vi "InClassProb9-TankIO.vi"() -> ()   [LabVIEW 2017]
panel:
  out "AI3 Heater":dbl(slide) scale=0.0..100.0
  out "AI2 Tank 2":dbl(slide) scale=0.0..10.0
  out "AI1 Tank 1":dbl(slide) scale=0.0..10.0
  out "AI0 Main":dbl(slide) scale=0.0..10.0
  out "AI3":dbl
  out "AI2":dbl
  out "AI1":dbl
  out "AI0":dbl
  in  "Spare":bool
  in  "CM":bool
  in  "PM":bool
  in  "HT-01":bool
  in  "DV-02":bool
  in  "DV-01":bool
  in  "FV-02":bool
  in  "FV-01":bool
  out "data[1]":bool
  out "data[0]":bool
  in  "stop":bool
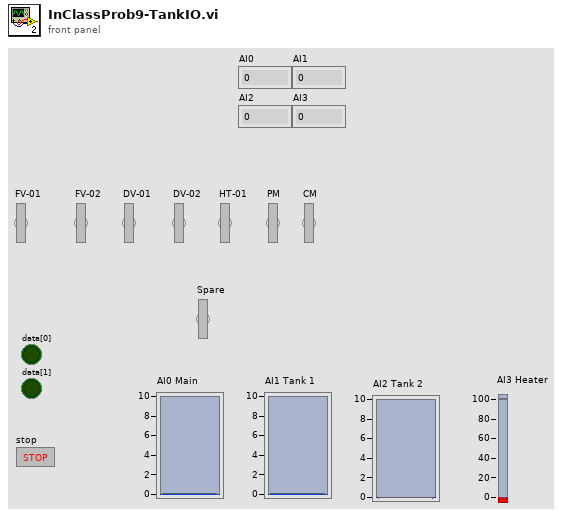
[diagram p1: front panel]
types:
  T1 = cluster{"data[0]":bool, "data[1]":bool, "data[2]":bool, "data[3]":bool, "data[4]":bool, "data[5]":bool, "data[6]":bool, "data[7]":bool, "data[8]":bool}
  T2 = cluster{"FV-01":bool, "FV-02":bool, "DV-01":bool, "DV-02":bool, "Spare":bool, "PM":bool, "CM":bool, "HT-01":bool}
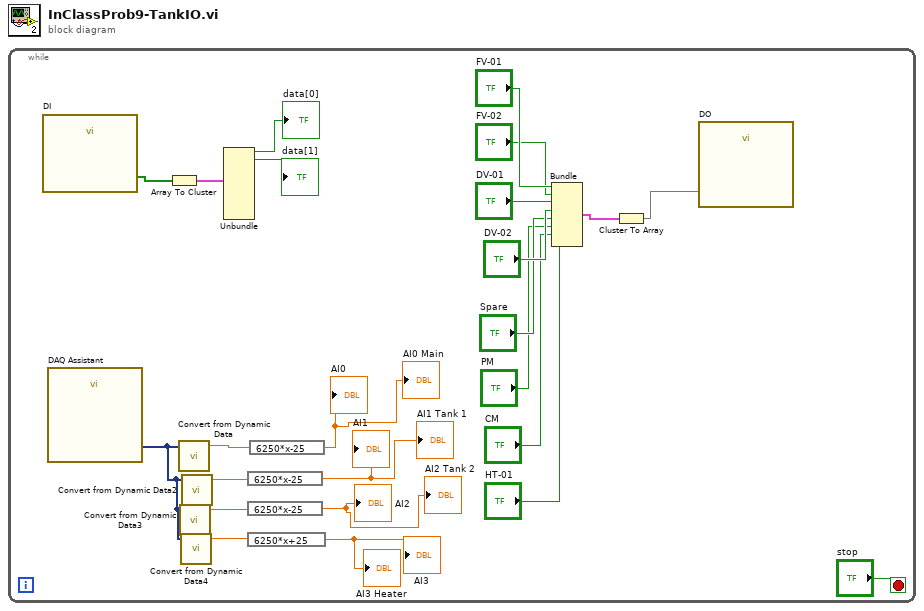
[diagram p0: block diagram]
diagram:
  n1 = while {
    stop <- "stop" stop-if-true
    n2 = call "DI"() -> ("data"=w23:bool[])  [unwired: 17 in, 2 out]
    n3 = call "DAQ Assistant"() -> ("data"=w9:dynamicdata)  [unwired: 17 in, 2 out]
    n4 = Array To Cluster(array=w23) -> (cluster=w22:T1)
    n5 = call "Convert from Dynamic Data"("Dynamic Data Type"=w9) -> ("Scalar"=w8:dbl)  [unwired: 3 in]
    n6 = call "Convert from Dynamic Data3"("Dynamic Data Type"=w9) -> ("Scalar"=w6:dbl)  [unwired: 3 in]
    n7 = call "Convert from Dynamic Data4"("Dynamic Data Type"=w9) -> ("Scalar"=w5:dbl)  [unwired: 3 in]
    n8 = call "Convert from Dynamic Data2"("Dynamic Data Type"=w9) -> ("Scalar"=w7:dbl)  [unwired: 3 in]
    n9 = Unbundle(w22) -> ("data[0]"=→"data[0]":bool, "data[1]"=→"data[1]":bool)  [unwired: 7 out]
    n10 = expression code="6250*x-25"(w7) -> (→"AI1" →"AI1 Tank 1":dbl)
    n11 = expression code="6250*x-25"(w6) -> (→"AI2" →"AI2 Tank 2":dbl)
    n12 = expression code="6250*x+25"(w5) -> (→"AI3" →"AI3 Heater":dbl)
    n13 = expression code="6250*x-25"(w8) -> (→"AI0" →"AI0 Main":dbl)
    n14 = Bundle("FV-01"="FV-01", "FV-02"="FV-02", "DV-01"="DV-01", "DV-02"="DV-02", "Spare"="Spare", "PM"="PM", "CM"="CM", "HT-01"="HT-01") -> (w11:T2)  [unwired: 1 in]
    n15 = Cluster To Array(cluster=w11) -> (array=w10:bool[])
    n16 = call "DO"("data"=w10) -> ()  [unwired: 17 in, 2 out]
  }
